vi "初始化+电阻单次采集.vi"(7 "通道号":i32, 11 "VISA引用句柄输入":refnum<visa-resource-name>) -> (0 "平均值":string, 2 "采集值+平均值":string[](array[string]))   [LabVIEW 2015]
uses:
  <vilib>/Analysis/baseanly.llb/Mean (DBL).vi
  Keithley 27XX/Keithley 27XX.lvlib
  <vilib>/Analysis/NI_AALBase.lvlib
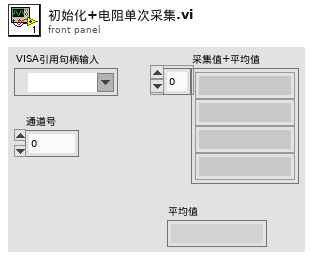
[diagram p1: front panel]
types:
  T1 = cluster{"Baud Rate (9600)":u32, "Flow Control (1: XON/XOFF)":u16, "Termination Char (0:CR)":u16}
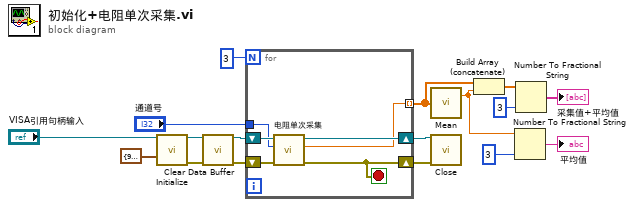
[diagram p0: block diagram]
diagram:
  n1 = call "Initialize.vi"("VISA resource name"="VISA引用句柄输入", "Serial Configuration"=T1 {"Baud Rate (9600)"=9600, "Flow Control (1: XON/XOFF)"=1, "Termination Char (0:CR)"=0}) -> ("VISA resource name out"=w11:refnum<visa-resource-name>, "error out"=w10:errorcluster)  [unwired: 12 in]
  n2 = call "Clear Data Buffer.vi"("VISA resource name"=w11, "error in (no error)"=w10) -> ("VISA resource name out"=w14:refnum<visa-resource-name>, "error out"=w15:errorcluster)  [unwired: 12 in]
  n3 = for {
    N: 3 -> [_]
    shift-right: [w18] -> w8
    shift-left: w15 -> [w23]
    shift-right: [w21] -> w9
    shift-left: w14 -> [w22]
    tunnel: [w20] -> w7 mode=indexing
    tunnel: "通道号" -> [w19]
    stop <- w18 stop-if-true
    n4 = call "电阻单次采集.vi"("错误输入（无错误）"=w23, "通道数"=w19, "VISA引用句柄输入"=w22) -> ("错误输出"=w18:errorcluster, "测量结果"=w20:dbl, "VISA引用句柄输出"=w21:refnum<visa-resource-name>)  [unwired: 5 in, 1 out]
  }
  n5 = call-poly <vilib>:"Mean.vi"("X"=w7) -> ("mean"=w4:dbl)  [unwired: 1 out]
  n6 = call "Close.vi"("VISA resource name"=w9, "error in (no error)"=w8) -> ()  [unwired: 13 in, 1 out]
  n7 = Build Array (concatenate)(w7, w4) -> (w6:dbl[])
  n8 = Number To Fractional String(number=w4, precision (6)=i16 3 ("精度(6)")) -> (F-format string=→"平均值":string)  [unwired: 2 in]
  n9 = Number To Fractional String(number=w6, precision (6)=i16 3 ("精度(6)")) -> (F-format string=→"采集值+平均值":string[])  [unwired: 2 in]
